vi "Move.vi"(10 "Array in":u64[](array[numeric]), 11 "Numeric":u64) -> (3 "Array out":u64[](array[numeric]))   [LabVIEW 2020]
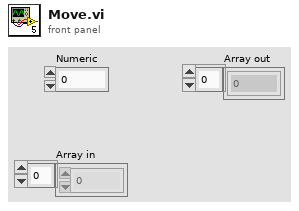
[diagram p1: front panel]
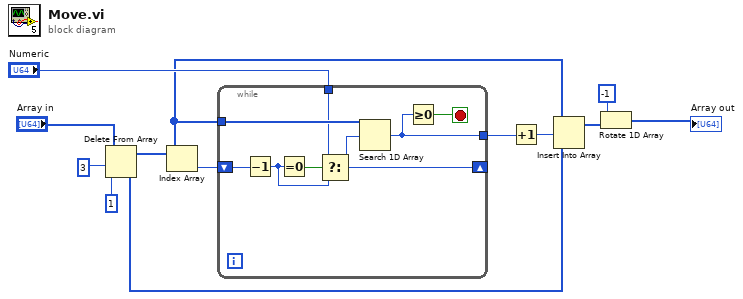
[diagram p0: block diagram]
diagram:
  n1 = Delete From Array(array="Array in", length=3, index=1) -> (deleted portion=w7:u64[], array with subset deleted=w4:u64[])
  n2 = Index Array(array=w4) -> (element=w8:u64)  [unwired: 1 in]
  n3 = while {
    tunnel: w4 -> [w17]
    shift-right: [w15] -> _
    shift-left: w8 -> [w20]
    tunnel: [w14] -> w5
    tunnel: "Numeric" -> [w13]
    stop <- w16 stop-if-true
    n4 = Decrement(x=w20) -> (x-1=w18:u64)
    n5 = Equal To 0?(x=w18) -> (x = 0?=w19:bool)
    n6 = Select(t=w13, s=w19, f=w18) -> (s? t:f=w15:u64)
    n7 = Search 1D Array(1D array=w17, element=w15) -> (index of element=w14:i32)  [unwired: 1 in]
    n8 = Greater Or Equal To 0?(x=w14) -> (x >= 0?=w16:bool)
  }
  n9 = Increment(x=w5) -> (x+1=w6:i32)
  n10 = Insert Into Array(array=w4, index=w6, new element=w7) -> (w9:u64[])
  n11 = Rotate 1D Array(1:w9, 2:-1 ("n")) -> (0:→"Array out":u64[])
